vi "test NtripClient.vi"() -> ()   [LabVIEW 2019]
uses:
  Ctrl/Ntrip_Account_db.ctl
  <vilib>/Instr/_visa.llb/VISA Configure Serial Port (Instr).vi
panel:
  in  "탭 컨트롤":enum32{"Main", "ref", "wireshark capture"}(tab)
  in  "Mount points":u16(ring) items=["FKP_V31", "SSRG", "VRS_V31", "VRS_V32"]
  out "RTCM recv":string
  in  "stop":bool
  in  "VISA resource name":refnum<visa-resource-name> caption="GNSS port"
  in  "정지":bool
  in  "baud rate (9600)":u32=9600 caption="rate"
  in  "write":bool
  out "station\nconn":bool
  out "server name":string
  out "mount points":string[](array[string])
  out "연결된 문자열":string
  out "링 텍스트.텍스트":string
  out "n1":i32
  out "n2":i32
  in  "Current Ntrip account":T1={"address"="gnss.eseoul.go.kr", "port "=2101, "id"="seoul", "pwd"="seoul", "ref pt"="YONS-RTCM32-M5"}
  in  "read bytes":i32=10000
  in  "t":string
  in  "s":bool
  # "fkp.ngii.go.kr"
  # "Test Ntrip Client"
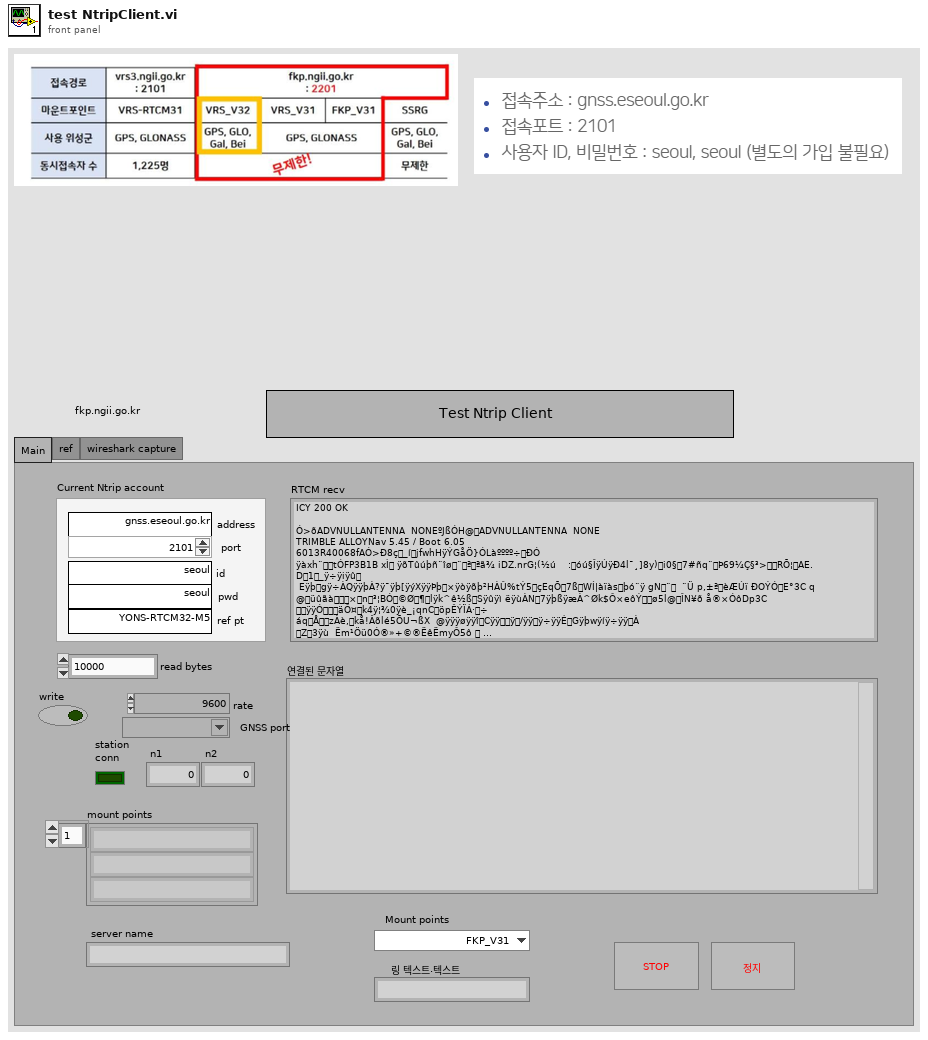
[diagram p1: front panel]
types:
  T1 = typedef "Ntrip_Account_db.ctl" = cluster{"address":string, "port ":u16, "id":string, "pwd":string, "ref pt":string}
  T2 = enum16{"Standard", "Buffered", "CRLF", "Immediate"}
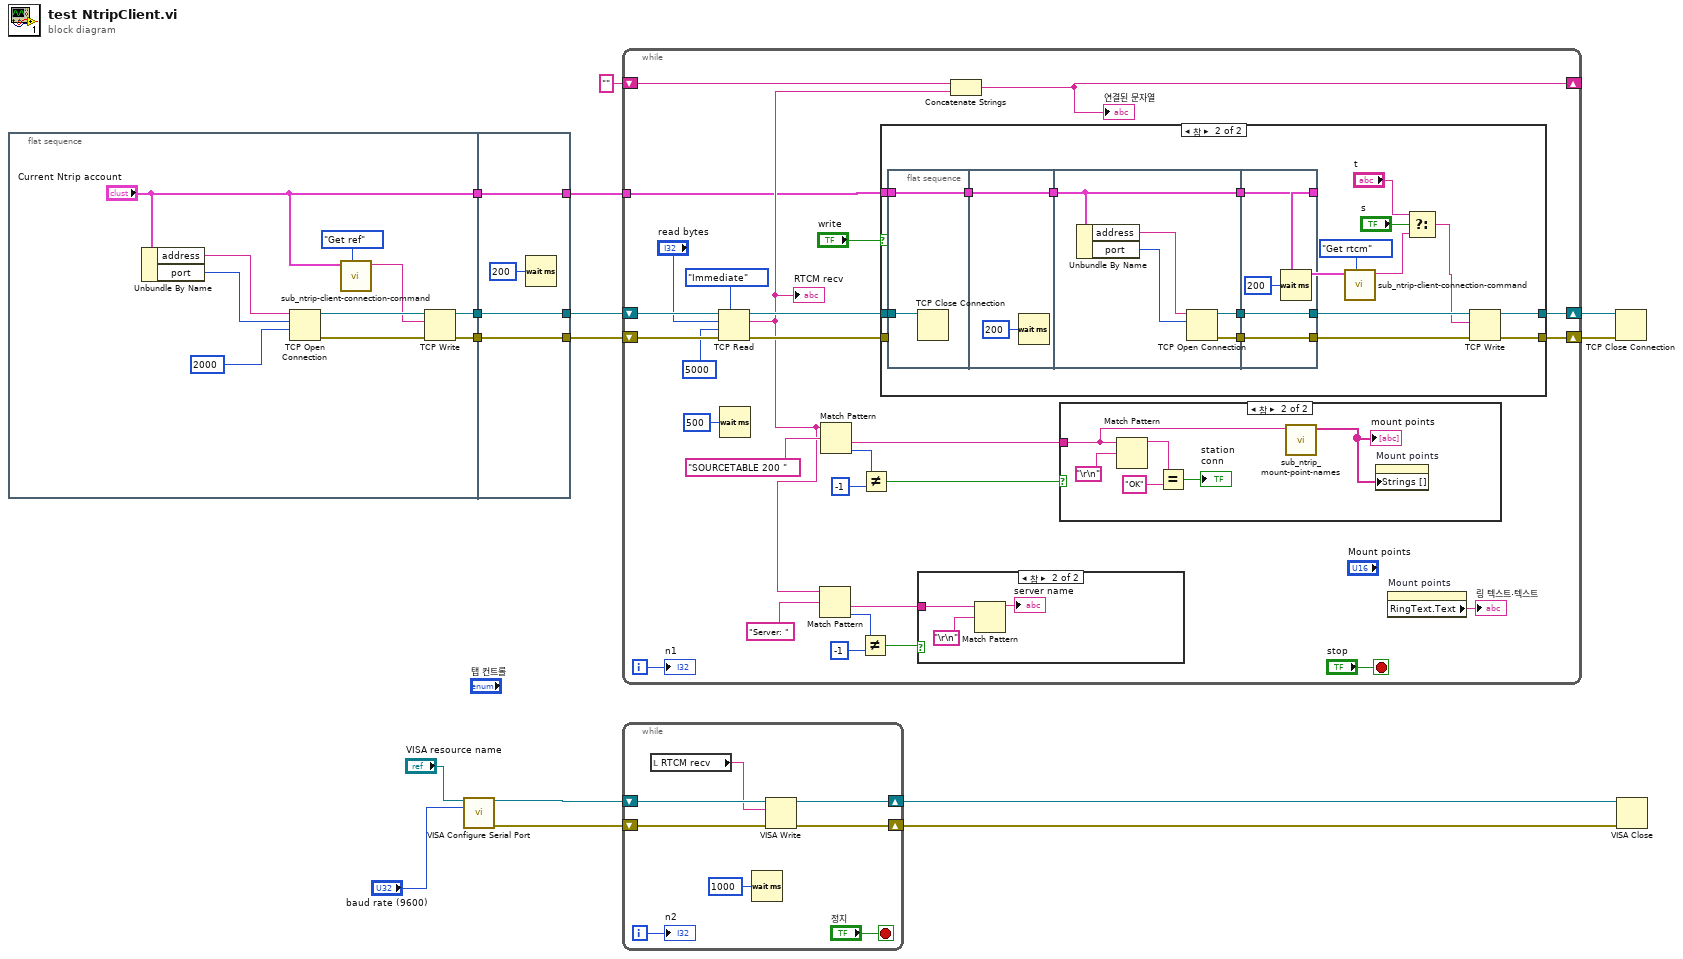
[diagram p0: block diagram]
diagram:
  n1 = flat-sequence {
    tunnel: [w23] -> w4
    tunnel: [w22] -> w3
    tunnel: ["Current Ntrip account"] -> w1
    tunnel: [w28] -> w12
    tunnel: [w29] -> w13
    tunnel: w4 -> [w29]
    tunnel: w3 -> [w28]
    tunnel: [w26] -> w2
    tunnel: w1 -> [w26]
    frame #0 {
      n2 = Unbundle By Name("Current Ntrip account") -> ("address"=w18:string, "port"=w17:u16)
      n3 = TCP Open Connection(address=w18, remote port or service name=w17, timeout ms (60000)=2000) -> (connection ID=w24:refnum<k5>, error out=w21:errorcluster)  [unwired: 2 in]
      n4 = call "sub_ntrip-client-connection-command.vi"("cmd"=enum16{"Get ref", "Get rtcm"}."Get ref", "Current Ntrip account"="Current Ntrip account") -> ("hex"=w20:string)  [unwired: 9 in]
      n5 = TCP Write(connection ID=w24, data in=w20, error in (no error)=w21) -> (connection ID out=w22:refnum<k5>, error out=w23:errorcluster)  [unwired: 1 in, 1 out]
    }
    frame #1 {
      n6 = Wait (ms)(milliseconds to wait=u32 200) -> ()  [unwired: 1 out]
    }
  }
  n7 = call-poly "VISA Configure Serial Port"("VISA resource name"="VISA resource name", "baud rate (9600)"="baud rate (9600)") -> ("VISA resource name out"=w11:refnum<visa-resource-name>, "error out"=w9:errorcluster)  [unwired: 12 in]
  n8 = while {
    shift-right: [w50] -> w14
    shift-left: w13 -> [w56]
    shift-right: [w49] -> w15
    shift-left: w12 -> [w55]
    shift-right: [w35] -> _
    shift-left: "" -> [w47]
    tunnel: w2 -> [w31]
    i -> [w33]
    stop <- "stop" stop-if-true
    n9 = TCP Read(connection ID=w55, bytes to read="read bytes", error in (no error)=w56, 7:T2."Immediate" ("mode (standard)"), 9:5000 ("타임아웃 ms (25000)")) -> (connection ID out=w51:refnum<k5>, data out=w36:string, error out=w52:errorcluster)
    "RTCM recv" <- w36
    n10 = Wait (ms)(milliseconds to wait=u32 500) -> ()  [unwired: 1 out]
    n11 = Match Pattern(string=w36, regular expression="Server: " ("정규식")) -> (after substring=w38:string, offset past match=w40:i32)  [unwired: 1 in, 2 out]
    n12 = Match Pattern(string=w36, regular expression="SOURCETABLE 200 " ("정규식")) -> (after substring=w45:string, offset past match=w43:i32)  [unwired: 1 in, 2 out]
    n13 = Not Equal?(x=w40, y=-1) -> (x != y?=w41:bool)
    n14 = Not Equal?(x=w43, y=-1) -> (x != y?=w42:bool)
    n15 = case shown="참" "write" {
      tunnel: w52 -> [w67 _]
      tunnel: w51 -> [w68 w82]
      tunnel: [w67 w85] -> w50
      tunnel: [w68 w84] -> w49
      tunnel: w31 -> [_ w79]
      frame False {
      }
      frame True {
        n16 = flat-sequence {
          tunnel: w82 -> [w87]
          tunnel: w79 -> [w86]
          tunnel: [w86] -> w78
          tunnel: w78 -> [w88]
          tunnel: [w88] -> w77
          tunnel: w77 -> [w90]
          tunnel: [w94] -> w71
          tunnel: [w93] -> w70
          tunnel: [w90] -> w69
          tunnel: [w96] -> w76
          tunnel: [w97] -> w80
          tunnel: [w98] -> w81
          tunnel: w71 -> [w98]
          tunnel: w70 -> [w97]
          tunnel: w69 -> [w96]
          frame #0 {
            n17 = TCP Close Connection(connection ID=w87) -> ()  [unwired: 2 in, 2 out]
          }
          frame #1 {
            n18 = Wait (ms)(milliseconds to wait=u32 200) -> ()  [unwired: 1 out]
          }
          frame #2 {
            n19 = Unbundle By Name(w90) -> ("address"=w92:string, "port"=w91:u16)
            n20 = TCP Open Connection(address=w92, remote port or service name=w91) -> (connection ID=w94:refnum<k5>, error out=w93:errorcluster)  [unwired: 3 in]
          }
          frame #3 {
            n21 = Wait (ms)(milliseconds to wait=u32 200) -> ()  [unwired: 1 out]
          }
        }
        n22 = call "sub_ntrip-client-connection-command.vi"("cmd"=enum16{"Get ref", "Get rtcm"}."Get rtcm", "Current Ntrip account"=w76) -> ("hex"=w74:string)  [unwired: 9 in]
        n23 = Select(t="t", s="s", f=w74) -> (s? t:f=w75:string)
        n24 = TCP Write(connection ID=w81, data in=w75, error in (no error)=w80) -> (connection ID out=w84:refnum<k5>, error out=w85:errorcluster)  [unwired: 1 in, 1 out]
      }
    }
    n25 = case shown="참" w41 {
      tunnel: w38 -> [_ w59]
      frame False {
      }
      frame True {
        n26 = Match Pattern(string=w59, regular expression="\r\n") -> (before substring=→"server name":string)  [unwired: 1 in, 3 out]
      }
    }
    n27 = Concatenate Strings(w47, w36) -> (w35:string)
    "연결된 문자열" <- w35
    n28 = case shown="참" w42 {
      tunnel: w45 -> [_ w62]
      frame False {
      }
      frame True {
        n29 = Match Pattern(string=w62, regular expression="\r\n") -> (before substring=w65:string)  [unwired: 1 in, 3 out]
        n30 = Equal?(x=w65, y="OK") -> (x = y?=→"station\nconn":bool)
        n31 = call "sub_ntrip_mount-point-names.vi"("ntrip str"=w62) -> ("mount points"=w61:string[])  [unwired: 10 in]
        "mount points" <- w61
        n32 = property on="Mount points" class="Ring (엄격한)"("Strings []"=w61) -> ()  [unwired: 2 in, 2 out]
      }
    }
    n33 = property on="Mount points" class="Ring (엄격한)"() -> ("RingText.Text"=→"링 텍스트.텍스트":string)  [unwired: 2 in, 2 out]
    "n1" <- w33
  }
  n34 = while {
    shift-right: [w105] -> w10
    shift-left: w11 -> [w106]
    shift-right: [w103] -> w8
    shift-left: w9 -> [w104]
    i -> [w99]
    stop <- "정지" stop-if-true
    n35 = local read "RTCM recv"() -> (w100:string)
    n36 = Wait (ms)(milliseconds to wait=u32 1000) -> ()  [unwired: 1 out]
    n37 = VISA Write(VISA resource name=w106, write buffer=w100, error in (no error)=w104) -> (VISA resource name out=w105:refnum<visa-resource-name>, error out=w103:errorcluster)  [unwired: 1 out]
    "n2" <- w99
  }
  n38 = TCP Close Connection(connection ID=w15, error in (no error)=w14) -> ()  [unwired: 1 in, 2 out]
  n39 = VISA Close(VISA resource name=w10, error in (no error)=w8) -> ()  [unwired: 1 out]
